vi "Write Tag.vi"(10 "Tag":string, 11 "Abs_Type in":refnum<class "Abs_Type.lvclass">) -> (3 "Abs_Type out":refnum<class "Abs_Type.lvclass">)   [LabVIEW 2021, in "Abs_Type.lvclass"]
uses:
  Abs_Type.lvclass
  Abs_Type.lvclass/Abs_Type.ctl
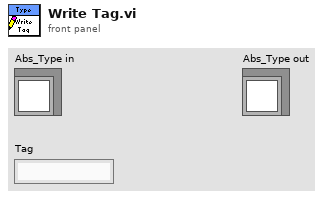
[diagram p1: front panel]
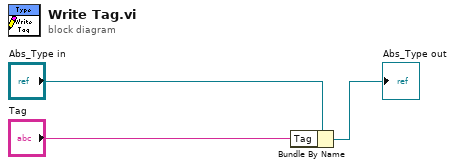
[diagram p0: block diagram]
diagram:
  n1 = Bundle By Name(cluster="Abs_Type in", "Tag"="Tag") -> (→"Abs_Type out":refnum<class "Abs_Type.lvclass">)
